vi "Print to temp file.vi"(8 "error in (no error)":errorcluster, 10 "VI reference":refnum<vi>, 11 "PrintToSingleFileHtml in":refnum<class "PrintToSingleFileHtml.lvclass">) -> (0 "error out":errorcluster, 2 "temp file path":path, 3 "PrintToSingleFileHtml out":refnum<class "PrintToSingleFileHtml.lvclass">)   [LabVIEW 2026, in "PrintToSingleFileHtml.lvclass"]
uses:
  PrintToSingleFileHtml.lvclass
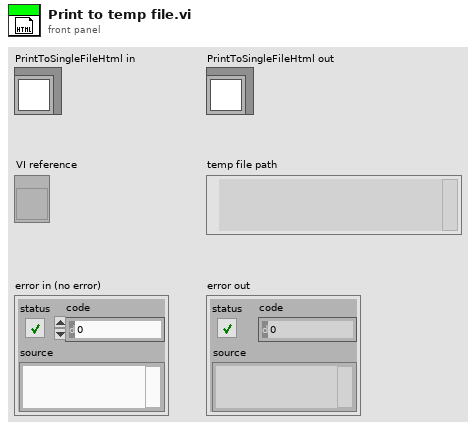
[diagram p1: front panel]
types:
  T1 = enum32{"Custom", "Standard", "Using Panel", "Using SubVI", "Complete"}
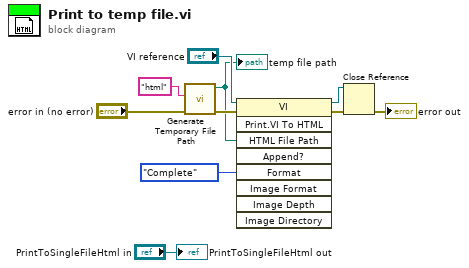
[diagram p0: block diagram]
diagram:
  n1 = call <vilib>:"Generate Temporary File Path.vi"("error in (no error)"="error in (no error)", "Temporary File Extension (tmp)"="html") -> ("error out"=w9:errorcluster, "Unique Temporary File Path"=w2:path)  [unwired: 8 in]
  "temp file path" <- w2
  n2 = invoke class="VI" method="Print.VI To HTML"(reference="VI reference", error in=w9, "HTML File Path"=w2, "Format"=T1."Complete") -> (reference out=w5:refnum<vi>, error out=w4:errorcluster)  [unwired: 5 in, 7 out]
  n3 = Close Reference(reference=w5, error in (no error)=w4) -> (error out=→"error out":errorcluster)
  "PrintToSingleFileHtml out" <- "PrintToSingleFileHtml in"
